vi "Watlow Write.vi"(0 "Adress":u8 format="%x", 1 "VISA resource name":refnum<visa-resource-name>="ASRL2::INSTR", 2 "Register":u32, 3 "Parameter":u32, 4 "error in (no error)":errorcluster) -> (5 "error out":errorcluster)   [LabVIEW 2009]
uses:
  <vilib>/Instr/_visa.llb/VISA Configure Serial Port (Instr).vi
panel:
  out "Serial Settings:Number of Bytes at Serial Port":u32
  out "Reg H":u32 format="%x"
  out "Reg L":u32 format="%x"
  out "unsigned byte array":u8[](array[numeric]) format="%x"
  out "Read buffer":string
  # "HEX"
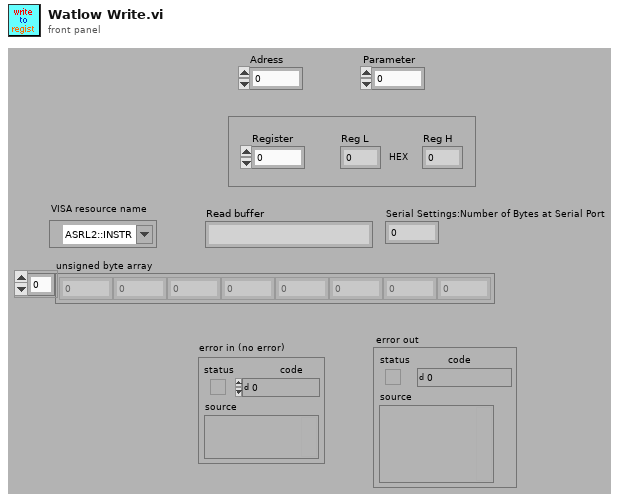
[diagram p1: front panel]
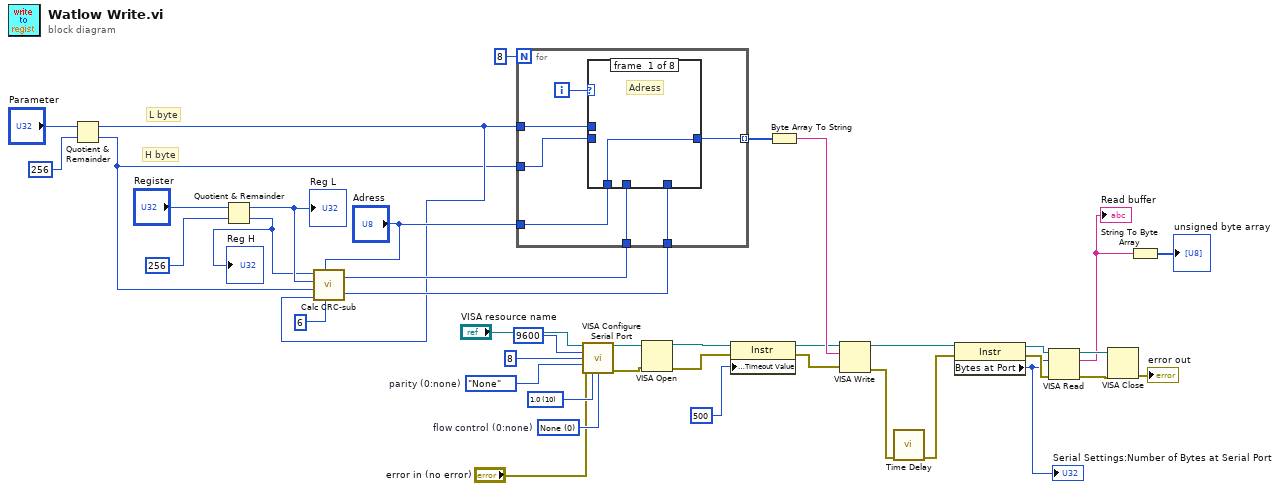
[diagram p0: block diagram]
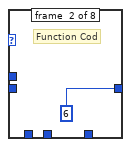
[diagram p2: hidden frame]
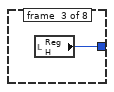
[diagram p3: hidden frame]
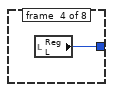
[diagram p4: hidden frame]
diagram:
  w22 = enum16{"None", "Odd", "Even", "Mark", "Space"}."None"  # parity (0:none)
  w23 = u16 0 items=["None"=0, "XON/XOFF"=1, "RTS/CTS"=2, "DTR/DSR"=4]  # flow control (0:none)
  w24 = u16 10 items=["1.0"=10, "1.5"=15, "2.0"=20] ("stop bits (10: 1 bit)")
  # "L byte"
  # "H byte"
  n1 = Quotient & Remainder(x="Parameter", y=u32 256) -> (x-y*floor(x/y)=w11:u32, floor(x/y)=w10:u32)
  n2 = Quotient & Remainder(x="Register", y=u32 256) -> (x-y*floor(x/y)=w7:u32, floor(x/y)=w6:u32)
  "Reg L" <- w7
  "Reg H" <- w6
  n3 = call "Calc CRC-sub.vi"("Command"=u8 6, "Adress"="Adress", "Data L"=w11, "Data H"=w10, "Reg L"=w7, "Reg H"=w6) -> ("L byte"=w16:u8, "H byte"=w15:u8)
  n4 = for {
    N: 8 -> [_]
    tunnel: [w46] -> w40 mode=indexing
    tunnel: w10 -> [w45]
    tunnel: w11 -> [w44]
    tunnel: w16 -> [w43]
    tunnel: w15 -> [w42]
    tunnel: "Adress" -> [w41]
    i -> [w47]
    n5 = case shown="0, Default" w47 {
      tunnel: [w48 u8 6 ("Command") w50 w51 w52 w53 w54 w55] -> w46
      tunnel: w45 -> [_ _ _ _ w52 _ _ _]
      tunnel: w44 -> [_ _ _ _ _ w53 _ _]
      tunnel: w43 -> [_ _ _ _ _ _ w54 _]
      tunnel: w42 -> [_ _ _ _ _ _ _ w55]
      tunnel: w41 -> [w48 _ _ _ _ _ _ _]
      frame #0 {
        # "Adress"
      }
      frame #1 {
        # "Function Cod"
      }
      frame #2 {
        n6 = local read "Reg H"() -> (w50:u32)
      }
      frame #3 {
        n7 = local read "Reg L"() -> (w51:u32)
      }
      frame #4 {
        # "Data H"
      }
      frame #5 {
        # "Data L"
      }
      frame #6 {
        # "CRC-L"
      }
      frame #7 {
        # "CRC-H"
      }
    }
  }
  n8 = call-poly "VISA Configure Serial Port"("VISA resource name"="VISA resource name", "baud rate (9600)"=u32 9600, "data bits (8)"=u16 8, "parity (0:none)"=w22, "error in (no error)"="error in (no error)", "stop bits (10: 1 bit)"=w24, "flow control (0:none)"=w23) -> ("VISA resource name out"=w36:refnum<visa-resource-name>, "error out"=w35:errorcluster)  [unwired: 7 out]
  n9 = VISA Open(error in (no error)=w35, VISA resource name=w36) -> (VISA resource name=w33:refnum<visa-resource-name>, error out=w32:errorcluster)  [unwired: 3 out]
  n10 = property class="Instr"(reference=w33, error in=w32, "General Settings:Timeout Value"=u32 500) -> (reference out=w31:refnum<visa-resource-name>, error out=w30:errorcluster)
  n11 = Byte Array To String(unsigned byte array=w40) -> (string=w37:string)
  n12 = VISA Write(VISA resource name=w31, write buffer=w37, error in (no error)=w30) -> (VISA resource name out=w21:refnum<visa-resource-name>, error out=w4:errorcluster)  [unwired: 1 out]
  n13 = call "Time Delay"("error in (no error)"=w4) -> ("error out"=w3:errorcluster)  [unwired: 1 in, 9 out]
  n14 = property class="Instr"(reference=w21, error in=w3) -> (reference out=w20:refnum<visa-resource-name>, error out=w5:errorcluster, "Bytes at Port"=w1:u32)
  "Serial Settings:Number of Bytes at Serial Port" <- w1
  n15 = VISA Read(VISA resource name=w20, byte count=w1, error in (no error)=w5) -> (VISA resource name out=w29:refnum<visa-resource-name>, read buffer=w19:string, error out=w28:errorcluster)  [unwired: 1 out]
  "Read buffer" <- w19
  n16 = VISA Close(VISA resource name=w29, error in (no error)=w28) -> (error out=→"error out":errorcluster)
  n17 = String To Byte Array(string=w19) -> (unsigned byte array=→"unsigned byte array":u8[])
